vi "Get Channel Mappings.vi"(8 "error in (no error)":errorcluster, 11 "Refnum in":T1) -> (0 "error out":errorcluster, 3 "Channel Mappings":cluster{string, string, "path capability":T2}[](array[cluster]) {"path capability" items=["Path Available"=1, "Path Exists"=2, "Path Unsupported"=3, "Resource in Use"=4, "Source Conflict"=5, "Channel Not Available"=6]})   [LabVIEW 2017]
uses:
  <vilib>/SLSC_Switch/Path Capability.ctl
  <vilib>/userdefined/High Color/SLSC_Switch/nislscslSession.ctl
  <vilib>/SLSC_Switch/SLSC Switch.lvlib
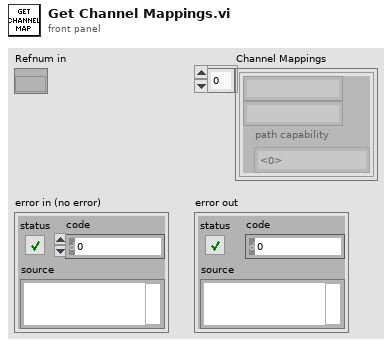
[diagram p1: front panel]
types:
  T1 = typedef "nislscslSession.ctl" = refnum<k20>
  T2 = typedef "SLSC Switch.lvlib/Path Capability.ctl" = i32
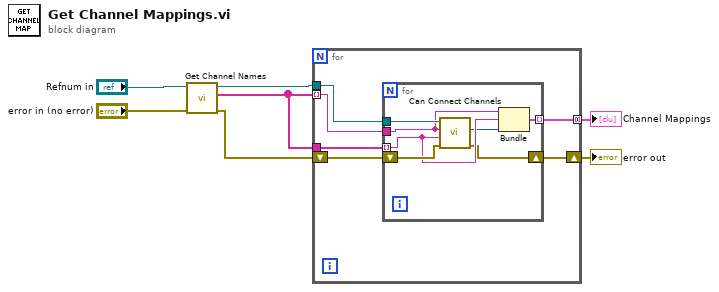
[diagram p0: block diagram]
diagram:
  n1 = call <vilib>:"Get Channel Names.vi"("error in (no error)"="error in (no error)", "session in"="Refnum in") -> ("error out"=w6:errorcluster, "channel names"=w4:string[], "session out"=w5:T1)  [unwired: 7 in]
  n2 = for {
    tunnel: w4 -> [w11] mode=indexing
    tunnel: w4 -> [w13]
    tunnel: w5 -> [w12]
    tunnel: [w9] -> w7 mode=concatenating
    shift-right: [w8] -> w1
    shift-left: w6 -> [w10]
    n3 = for {
      tunnel: w13 -> [w17] mode=indexing
      tunnel: w12 -> [w20]
      tunnel: w11 -> [w18]
      tunnel: [w15] -> w9 mode=indexing
      shift-right: [w14] -> w8
      shift-left: w10 -> [w19]
      n4 = call <vilib>:"Can Connect Channels.vi"("error in (no error)"=w19, "channel 2"=w17, "channel 1"=w18, "session in"=w20) -> ("error out"=w14:errorcluster, "path capability"=w16:T2)  [unwired: 5 in, 1 out]
      n5 = Bundle(w18, w17, "path capability"=w16) -> (w15:cluster{string, string, "path capability":T2})  [unwired: 1 in]
    }
  }
  "Channel Mappings" <- w7
  "error out" <- w1
